vi "D-O Module (Main) Try Again.vi"(7 "Name of Parent Panel":string="Main.vi", 9 "New Center Coords":T1={"Horizontal"=470, "Vertical"=200}, 10 "Config":variant, 11 "Main UI Message Queue":refnum<queue>) -> ()   [LabVIEW 2018]
uses:
  support/Message Queue/Message Cluster.ctl
  <vilib>/Utility/miscctls.llb/LVPoint32TypeDef.ctl
  controls/UI State.ctl
  controls/UI Data.ctl
  D-O Module Config Cluster.ctl
  Valve Clusters.ctl
  D-O Module Settings Cluster.ctl
  D-O Device Settings Cluster.ctl
  VICI Electronic Actuator/VICI Electronic Actuator Settings.ctl
  D-O Module State Cluster.ctl
  Measure Instrument/State Enum.ctl
  D-O Module Display.ctl
  Sequencing/Squence Update Cluster.ctl
  support/Message Queue/Enqueue Message (Single).vi
  support/Message Queue/Message Queue.lvlib
  support/Support Library.lvlib
  support/Command Log VIs/Command Logging.lvlib
  D-O Module.lvlib
  Sequencing/Sequencing Library.lvlib
  Measure Instrument/Feed Module Engine.lvlib
  support/User Event - Stop/User Event - Stop.lvlib
  D-O Settings Dialog.vi
  Measure Instrument/D-O Module Engine.lvlib
  DIO Valve/VICI Electronic Actuator.lvlib
panel:
  out "Sequence Started":bool
  out "ScanCode":i16
  in  "Settings Button":bool
  in  "Exit":bool
  out "Ring":u16(ring)=2
  out "Status":string
  out "Log File path":path
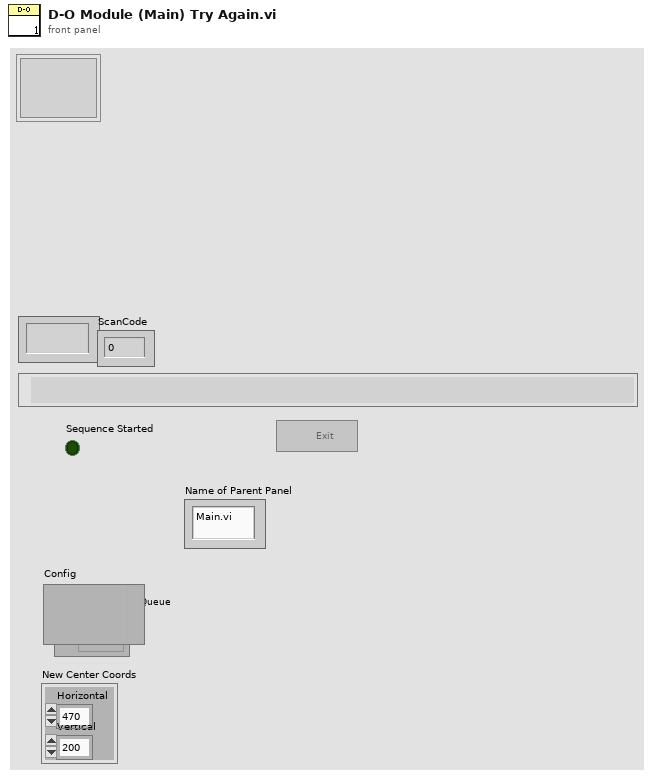
[diagram p1: front panel]
types:
  T1 = typedef "LVPoint32TypeDef.ctl" = cluster{"Horizontal":i32, "Vertical":i32}
  T2 = typedef "D-O Module.lvlib/D-O Module State Cluster.ctl" = cluster{"D-O Module Config":T3, "State":T8, "Start Time":timestamp, "Current Time":timestamp, "First Iteration":bool, "Data":cluster{"Valve State":T5}, "Process Name":string, "Queue Name":string, "Program On?":bool}
  T3 = typedef "D-O Module.lvlib/D-O Module Config Cluster.ctl" = cluster{"GUID":string, "Drop Coords":T1, "Process Name":string, "User name":string, "Queue Name":string, "Settings":T4, "Load Count":i32}
  T4 = typedef "D-O Module.lvlib/Valve Clusters.ctl" = cluster{"Valve Settings":T5, "Valve Type":enum16{"Default", "Digital Output Valve", "VICI Electronic Actuator"}, "Time On (Sec)":dbl, "Time Off (Sec)":dbl, "Run?":bool}
  T5 = typedef "D-O Module.lvlib/D-O Module Settings Cluster.ctl" = cluster{"D-O Settings":T6, "VICI Electronic Actuator":T7}
  T6 = typedef "D-O Module.lvlib/D-O Device Settings Cluster.ctl" = cluster{"DAQmx Task Name":refnum<k21>, "Output Channel":u16, "Output Channel Names":string[]}
  T7 = typedef "VICI Electronic Actuator.lvlib/VICI Electronic Actuator Settings.ctl" = cluster{"VISA resource name":refnum<visa-resource-name>, "Mode":enum16{"Two Positions With Stops", "Two Positions Without Stops", "Mutiposition"}, "Simulated":bool}
  T8 = typedef "Feed Module.lvlib/Feed Module Engine.lvlib/State Enum.ctl" = enum16{"Measuring", "Idle", "Paused"}
  T9 = typedef "UI Data.ctl" = cluster{"Start Ref":refnum<vi>, "Trigger Ref":refnum<vi>, "Stop Ref":refnum<vi>, "Settings Ref":refnum<vi>, "Status Ref":refnum<vi>, "Exit Ref":refnum<vi>, "Data Ref":refnum<vi>}
  T10 = typedef "UI State.ctl" = enum16{"Idle", "Acquiring and Logging", "Waiting for Exit", "Waiting for Exit (Acq Stopped)", "Waiting for Exit (Log Stopped)", "Waiting for Stop", "Waiting for Stop (Acq Stopped)", "Waiting for Stop (Log Stopped)"}
  T11 = typedef "D-O Module.lvlib/All Message Queues.ctl" = cluster{"Engine":refnum<queue>, "D-O UI":refnum<queue>, "D-O Engine":refnum<queue>, "D-O Display":refnum<queue>}
  T12 = typedef "Sequencing Library.lvlib/Squence Update Cluster.ctl" = cluster{"Auto?":bool, "Manual Entry":dbl, "Setpoint":dbl}
  T13 = enum8{"Enabled", "Disabled", "Disabled and Grayed Out"}
  T14 = typedef "D-O Module.lvlib/D-O Module Display.ctl" = cluster{"D-O State ":u16, "Cycle Period":dbl}
  T15 = cluster{"Shift":bool, "Ctrl":bool, "Alt":bool, "Cmd":bool, "Opt":bool}
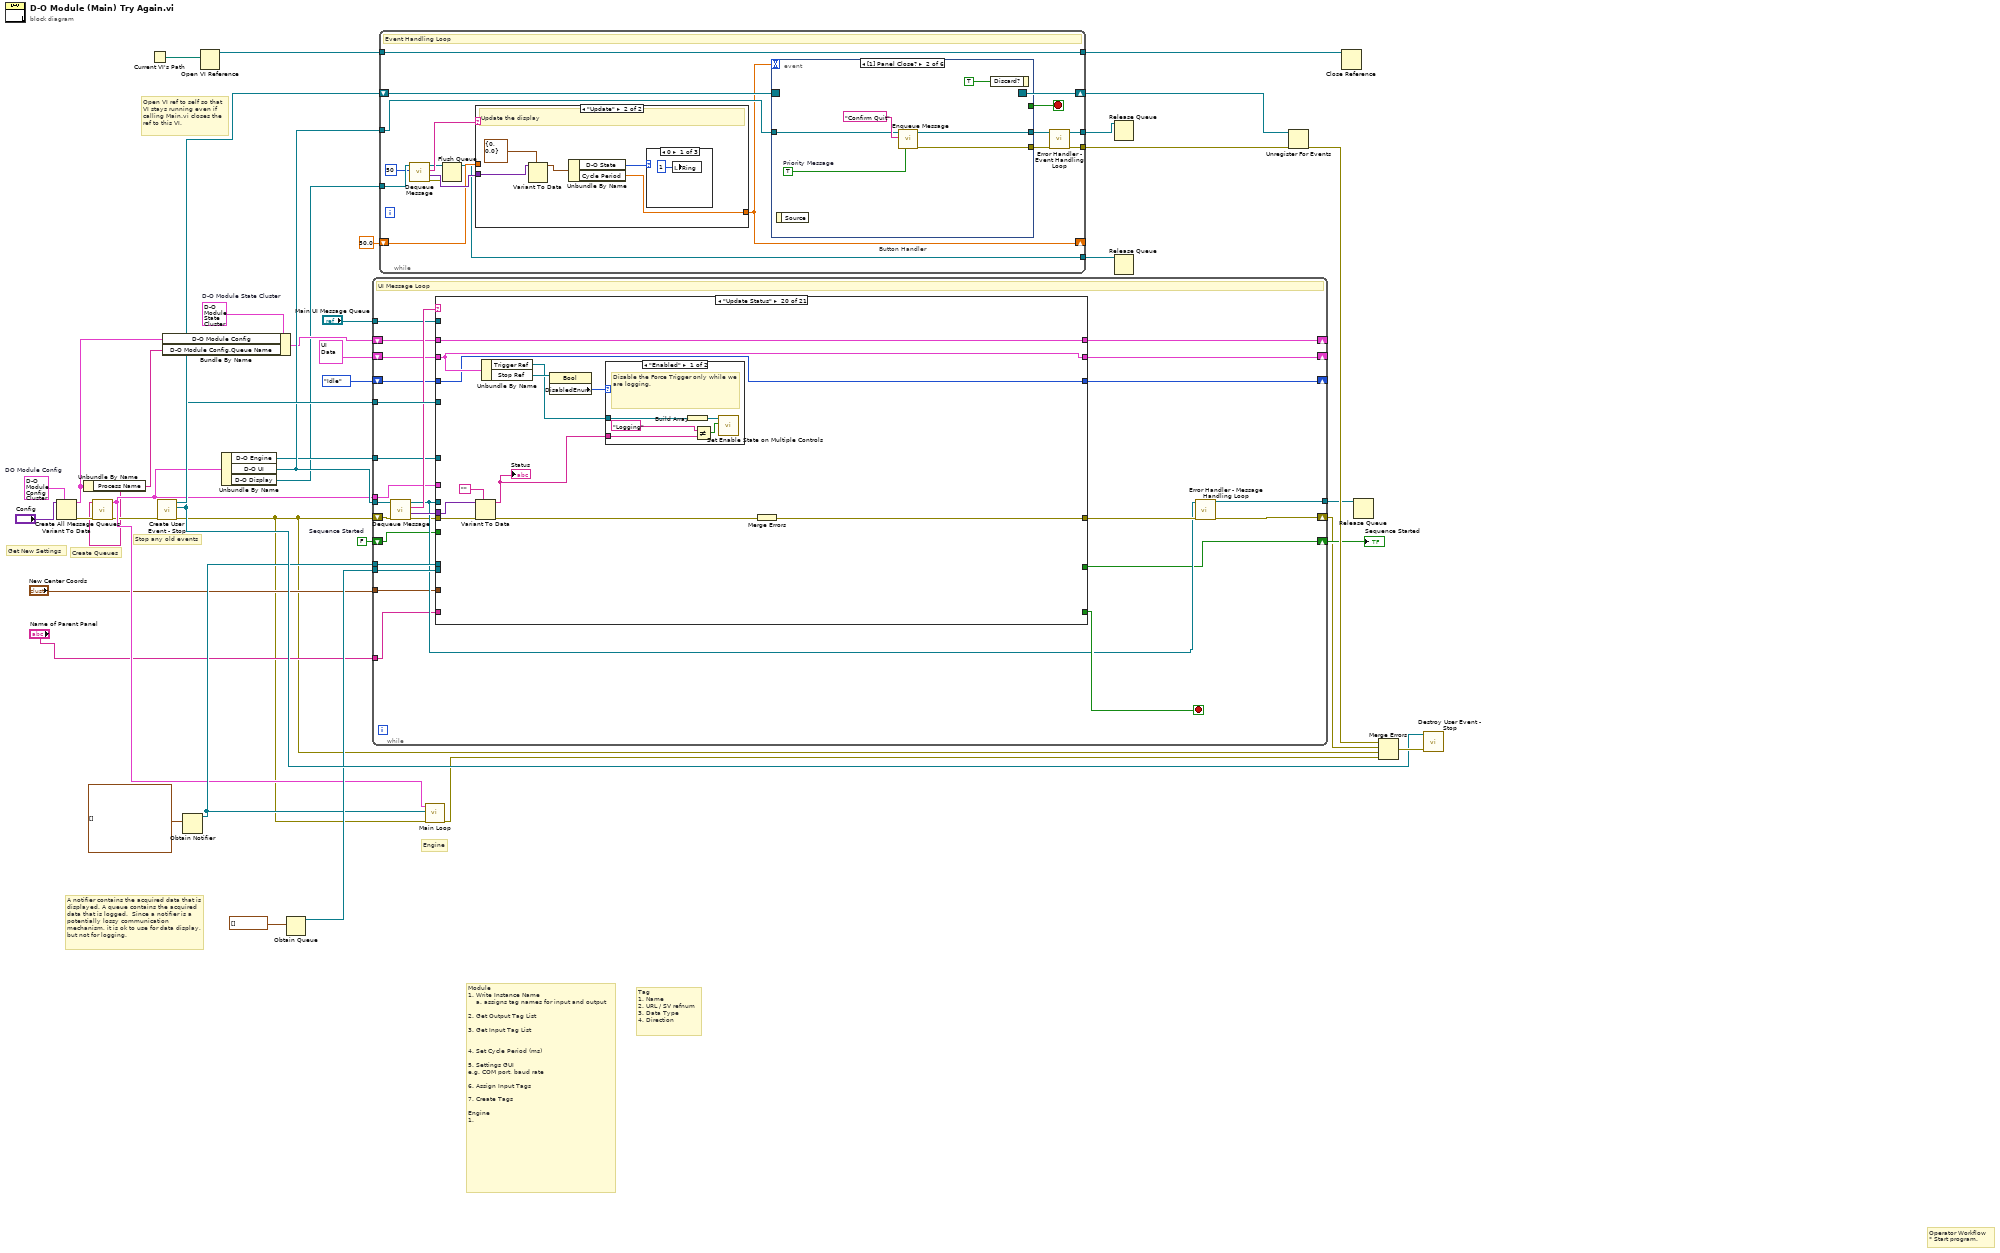
[diagram p0: block diagram]
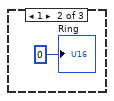
[diagram p3: hidden frame]
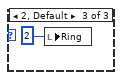
[diagram p4: hidden frame]
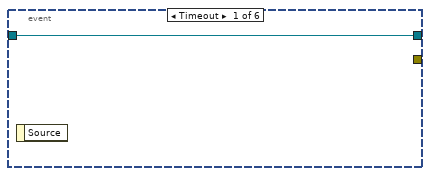
[diagram p5: hidden frame]
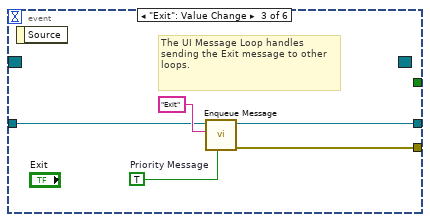
[diagram p6: hidden frame]
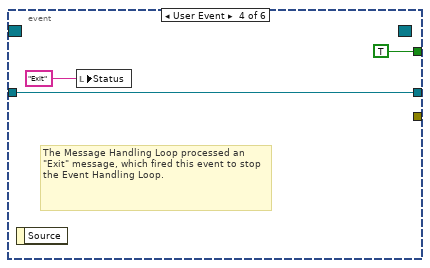
[diagram p7: hidden frame]
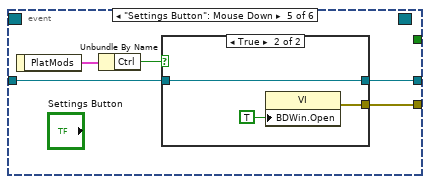
[diagram p8: hidden frame]
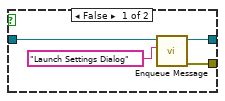
[diagram p9: hidden frame]
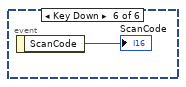
[diagram p10: hidden frame]
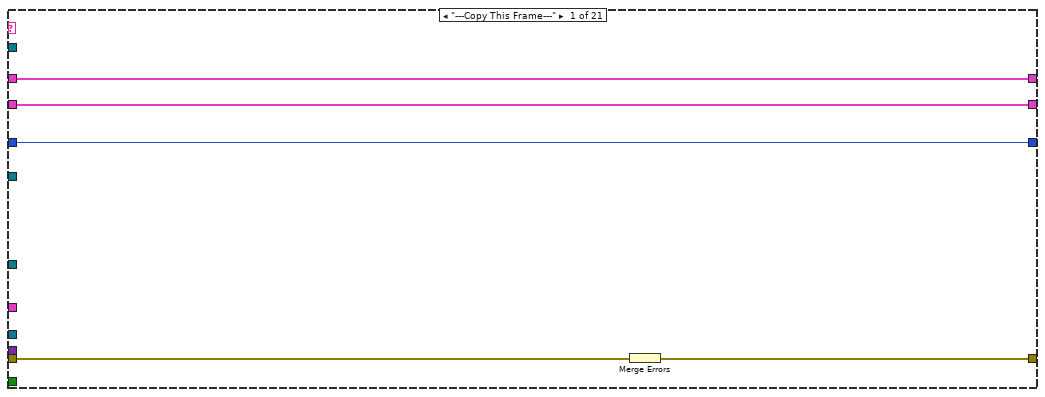
[diagram p11: hidden frame]
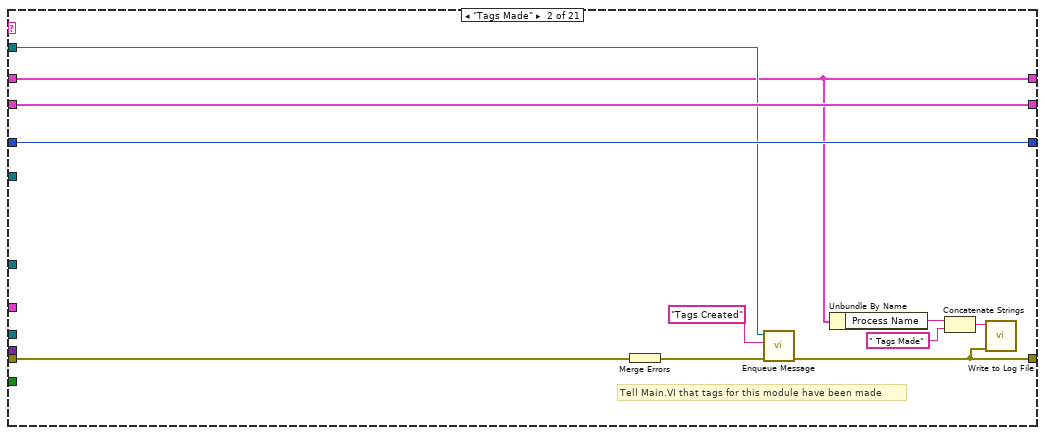
[diagram p12: hidden frame]
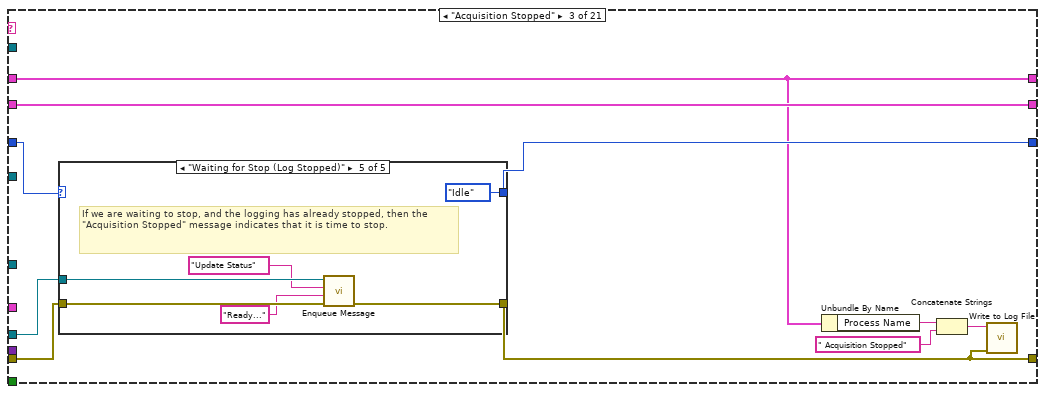
[diagram p13: hidden frame]
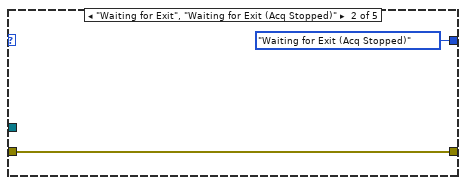
[diagram p15: hidden frame]
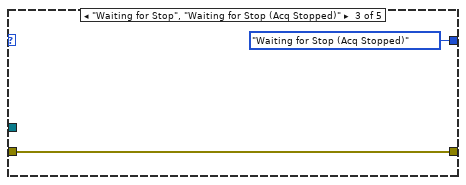
[diagram p16: hidden frame]
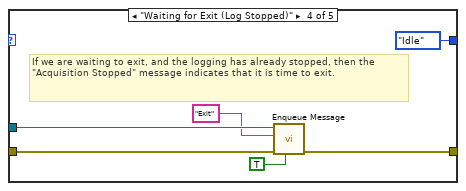
[diagram p17: hidden frame]
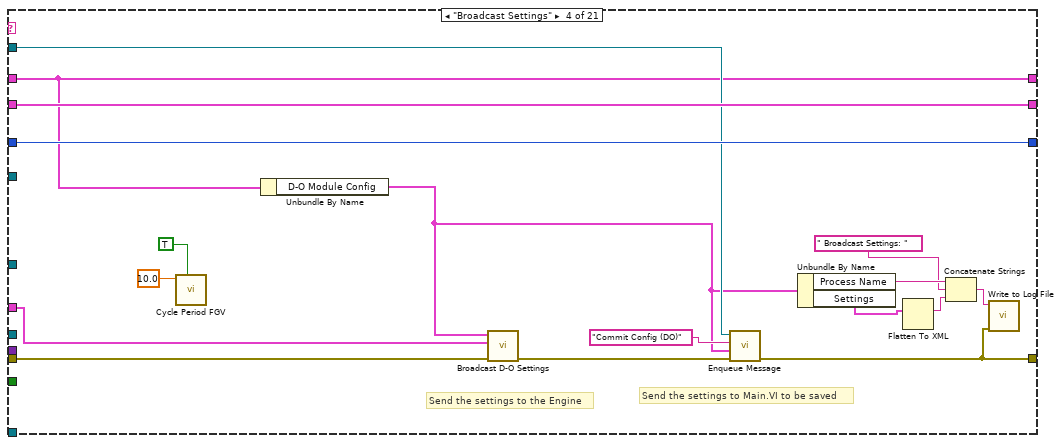
[diagram p18: hidden frame]
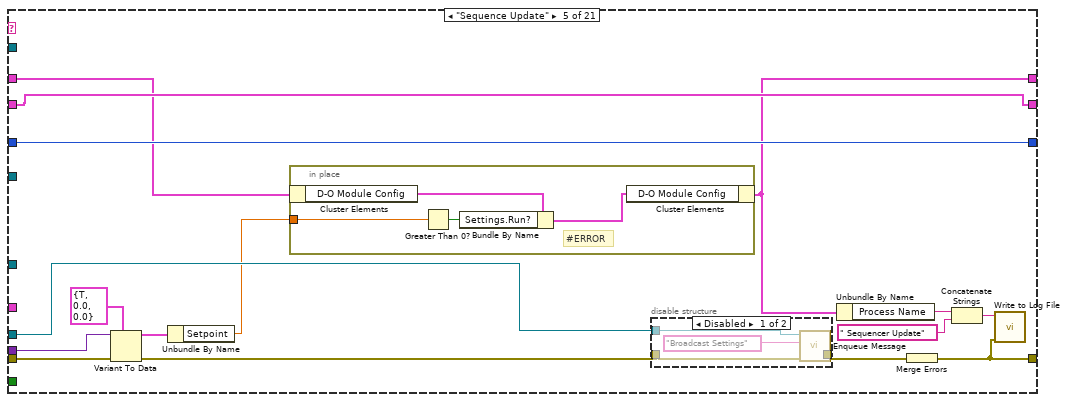
[diagram p19: hidden frame]
diagram:
  w19 = T2 {"D-O Module Config"={"GUID"="", "Drop Coords"={"Horizontal"=0, "Vertical"=0}, "Process Name"="", "User name"="", "Queue Name"="", "Settings"={"Valve Settings"={"D-O Settings"={"DAQmx Task Name"="", "Output Channel"=0, "Output Channel Names"=[]}, "VICI Electronic Actuator"={"VISA resource name"="", "Mode"=enum."Two Positions With Stops", "Simulated"=FALSE}}, "Valve Type"=enum."Digital Output Valve", "Time On (Sec)"=0.0, "Time Off (Sec)"=0.0, "Run?"=FALSE}, "Load Count"=0}, "State"=enum."Idle", "Start Time"=timestamp(0 s since 1904-01-01), "Current Time"=timestamp(0 s since 1904-01-01), "First Iteration"=FALSE, "Data"={"Valve State"={"D-O Settings"={"DAQmx Task Name"="", "Output Channel"=0, "Output Channel Names"=[]}, "VICI Electronic Actuator"={"VISA resource name"="", "Mode"=enum."Two Positions With Stops", "Simulated"=FALSE}}}, "Process Name"="", "Queue Name"="", "Program On?"=FALSE}  # D-O Module State Cluster
  w11 = T3 {"GUID"="", "Drop Coords"={"Horizontal"=0, "Vertical"=0}, "Process Name"="", "User name"="", "Queue Name"="", "Settings"={"Valve Settings"={"D-O Settings"={"DAQmx Task Name"="", "Output Channel"=0, "Output Channel Names"=[]}, "VICI Electronic Actuator"={"VISA resource name"="", "Mode"=enum."Two Positions With Stops", "Simulated"=FALSE}}, "Valve Type"=enum."Default", "Time On (Sec)"=0.0, "Time Off (Sec)"=0.0, "Run?"=FALSE}, "Load Count"=0}  # DO Module Config
  w12 = FALSE  # Sequence Started
  # "Stop any old events"
  # "Create Queues"
  # "Get New Settings"
  # "Open VI ref to self so that\nVI stays running even if\ncalling Main.vi closes the\nref to this VI."
  # "Engine"
  # "Operator Workflow\n* Start program."
  # "Module \n1. Write Instance Name\n    a. assigns tag names for input and output\n\n2. Get Output Tag List\n\n3. Get Input Tag List\n\n\n4. Set Cycle Period (ms)\n\n5. Settings GUI\ne.g. COM port, baud rate\n\n6. Assign Input Tags\n\n7. Create Tags\n\nEngine\n1."
  # "Tag\n1. Name\n2. URL / SV refnum\n3. Data Type\n4. Direction"
  # "A notifier contains the acquired data that is displayed. A queue contains the acquired data that is logged.  Since a notifier is a potentially lossy communication mechanism, it is ok to use for data display, but not for logging."
  n1 = Variant To Data(type=w11, Variant="Config") -> (data=w10:T3, error out=w9:errorcluster)  [unwired: 1 in]
  n2 = Unbundle By Name(w10) -> ("Process Name"=w6:string)
  n3 = call "Create All Message Queues.vi"("error in (no error)"=w9, "Process Name"=w6) -> ("error out"=w8:errorcluster, "Message Queues"=w16:T11)  [unwired: 8 in]
  n4 = Current VI's Path() -> (path=w22:path)
  n5 = call "Create User Event - Stop.vi"("error in (no error)"=w8) -> ("error out"=w7:errorcluster, "User Event - Stop"=w36:refnum<user-event>, "Stop Event Registration Refnum"=w37:refnum<event-registration>)  [unwired: 8 in]
  n6 = Bundle By Name(cluster=w19, "D-O Module Config"=w10, "D-O Module Config.Queue Name"=w6) -> (w21:T2)
  n7 = Obtain Notifier(notification data type=waveform(dbl)[] []) -> (notifier out=w25:refnum<notifier>)  [unwired: 3 in, 2 out]
  n8 = Open VI Reference(vi path=w22) -> (vi reference=w23:refnum<vi>)  [unwired: 5 in, 1 out]
  n9 = Unbundle By Name(w16) -> ("D-O Engine"=w28:refnum<queue>, "D-O UI"=w32:refnum<queue>, "D-O Display"=w18:refnum<queue>)
  n10 = Obtain Queue(element data type=waveform(dbl)[] []) -> (queue out=w27:refnum<queue>)  [unwired: 4 in, 2 out]
  n11 = while {
    tunnel: w32 -> [w60]
    tunnel: w36 -> [w64]
    shift-right: [w54] -> w2
    shift-left: w7 -> [w63]
    shift-right: [w41] -> _
    shift-left: w21 -> [w48]
    shift-right: [w58] -> _
    shift-left: T9 {"Start Ref"=refnum, "Trigger Ref"=refnum, "Stop Ref"=refnum, "Settings Ref"=refnum, "Status Ref"=refnum, "Exit Ref"=refnum, "Data Ref"=refnum} ("Measurement UI Controls") -> [w59]
    tunnel: w25 -> [w57]
    tunnel: w27 -> [w56]
    shift-right: [w51] -> _
    shift-left: UI_State."Idle" ("UI State") -> [w52]
    tunnel: w28 -> [w50]
    tunnel: "Main UI Message Queue" -> [w47]
    tunnel: w16 -> [w46]
    tunnel: "New Center Coords" -> [w45]
    tunnel: "Name of Parent Panel" -> [w44]
    shift-right: [w43] -> w13
    shift-left: w12 -> [w42]
    tunnel: [w40] -> w1
    stop <- w65 stop-if-true
    # "UI Message Loop"
    n12 = call "Dequeue Message.vi"("error in (no error)"=w63, "Message Queue"=w60) -> ("error out"=w49:errorcluster, "Message Data"=w61:variant, "Message"=w62:string, "dup Message Queue"=w53:refnum<queue>)  [unwired: 6 in]
    n13 = case "Message Cases" shown="\"Update Status\"" w62 {
      selector: w62 -> [_ _ _ _ _ _ _ _ _ _ _ _ _ _ _ _ _ _ _ _ w487]
      tunnel: w53 -> [_ _ w87 _ w139 w158 _ w216 w231 w258 _ w292 w311 w317 w353 w384 _ _ w444 _ _]
      tunnel: w49 -> [w70 w81 w88 w123 w138 w157 w184 w197 w235 w262 w277 w287 w309 w319 w351 w383 w410 w421 w446 w479 _]
      tunnel: [w69 w75 w86 w116 w129 w152 w185 w191 w225 w237 w277 w282 w305 w318 w342 w372 w414 w426 w441 w480 w486] -> w55
      tunnel: [_ _ _ _ _ _ _ _ _ TRUE _ _ _ _ _ _ _ _ _ _ _] -> w65
      tunnel: w61 -> [_ _ _ _ w140 _ w187 _ w234 w246 _ _ _ _ _ _ _ _ _ w478 _]
      tunnel: w64 -> [_ _ _ _ _ _ _ _ _ w261 _ _ _ _ _ _ _ _ _ _ _]
      tunnel: w48 -> [w66 w71 w82 w120 w128 w151 w182 w195 w222 w238 w268 w278 w300 w316 w347 w379 w408 w422 w448 w469 w492]
      tunnel: w59 -> [w68 w80 w91 w126 w141 w160 w189 w213 w236 w259 w276 w288 w313 w322 w348 w380 w413 w431 w464 w475 w497]
      tunnel: [w68 w80 w91 w126 w141 w160 w189 w213 w236 w259 w275 w288 w313 w322 w348 w380 w413 w431 w464 w475 w497] -> w58
      tunnel: w57 -> [_ _ _ _ _ _ _ _ _ w257 _ _ _ _ _ _ _ _ _ _ _]
      tunnel: w56 -> [_ _ _ _ _ _ _ _ _ w253 _ _ _ _ _ _ _ _ _ _ _]
      tunnel: w52 -> [w67 w79 w90 w125 w142 w159 w183 w202 w226 _ _ _ w312 w321 _ _ _ _ w453 w470 w496]
      tunnel: [w67 w79 w89 w125 w142 w156 w183 w203 w226 UI_State."Idle" ("UI State") UI_State."Idle" ("UI State") UI_State."Idle" ("UI State") w312 w320 UI_State."Acquiring and Logging" ("UI State") UI_State."Acquiring and Logging" ("UI State") UI_State."Acquiring and Logging" ("UI State") UI_State."Acquiring and Logging" ("UI State") w454 w470 w496] -> w51
      tunnel: w50 -> [_ _ _ _ _ _ _ w201 _ w245 _ _ _ _ _ _ w411 w429 w452 _ _]
      tunnel: w47 -> [_ w76 _ w122 _ _ _ _ _ w247 _ _ _ _ _ _ _ _ _ _ _]
      tunnel: [w66 w71 w82 w120 w127 w151 w182 w190 w222 w238 w268 w278 w301 w316 w341 w369 w408 w422 w437 w469 w492] -> w41
      tunnel: w46 -> [_ _ _ w118 _ _ _ _ _ _ _ _ w307 _ _ _ _ _ _ _ _]
      tunnel: w45 -> [_ _ _ _ _ _ _ _ _ _ _ w285 _ _ _ _ _ _ _ _ _]
      tunnel: w44 -> [_ _ _ _ _ _ _ _ _ _ _ w284 _ _ _ _ _ _ _ _ _]
      tunnel: [_ _ _ _ _ _ _ _ _ _ _ _ _ _ _ w377 _ _ _ _ _] -> w43
      tunnel: w42 -> [_ _ _ _ _ _ _ _ _ _ _ _ _ _ _ w373 _ _ _ _ _]
      frame "---Copy This Frame---" {
        # "Duplicate this frame when creating new messages.  Change this comment in the duplicated frame to describe this message."
        n14 = Merge Errors(w70) -> (w69:errorcluster)
      }
      frame "Tags Made" {
        # "Tell Main.VI that tags for this module have been made"
        # "Duplicate this frame when creating new messages.  Change this comment in the duplicated frame to describe this message."
        n15 = Merge Errors(w81) -> (w77:errorcluster)
        n16 = call-poly "Enqueue Message.vi"("error in (no error)"=w77, "Message"="Tags Created", "Message Queue"=w76) -> ("error out"=w75:errorcluster)  [unwired: 7 in, 1 out]
        n17 = Unbundle By Name(w71) -> ("Process Name"=w74:string)
        n18 = Concatenate Strings(w74, " Tags Made" ("text")) -> (w72:string)
        n19 = call "Write to Log File.vi"("error in"=w75, "text"=w72) -> ()  [unwired: 9 in, 1 out]
      }
      frame "Acquisition Stopped" {
        # "Logic for determining what action to take when the acquisition has stopped."
        n20 = case shown="\"Waiting for Stop (Log Stopped)\"" w90 {
          selector: w90 -> [w93 _ _ _ _]
          tunnel: [w93 UI_State."Waiting for Exit (Acq Stopped)" ("UI State") UI_State."Waiting for Stop (Acq Stopped)" ("UI State") UI_State."Idle" ("UI State") UI_State."Idle" ("UI State")] -> w89
          tunnel: w88 -> [w92 w94 w96 w102 w108]
          tunnel: [w92 w94 w96 w101 w107] -> w86
          tunnel: w87 -> [_ _ _ w100 w106]
          frame Default {
          }
          frame "Waiting for Exit", "Waiting for Exit (Acq Stopped)" {
          }
          frame "Waiting for Stop", "Waiting for Stop (Acq Stopped)" {
          }
          frame "Waiting for Exit (Log Stopped)" {
            # "If we are waiting to exit, and the logging has already stopped, then the \"Acquisition Stopped\" message indicates that it is time to exit."
            n21 = call-poly "Enqueue Message.vi"("Priority Message? (F)"=TRUE, "error in (no error)"=w102, "Message"="Exit", "Message Queue"=w100) -> ("error out"=w101:errorcluster)  [unwired: 6 in, 1 out]
          }
          frame "Waiting for Stop (Log Stopped)" {
            # "If we are waiting to stop, and the logging has already stopped, then the \"Acquisition Stopped\" message indicates that it is time to stop."
            n22 = call-poly "Enqueue Message.vi"("error in (no error)"=w108, "Message Data"="Ready..." ("Message"), "Message"="Update Status", "Message Queue"=w106) -> ("error out"=w107:errorcluster)  [unwired: 6 in, 1 out]
          }
        }
        n23 = Unbundle By Name(w82) -> ("Process Name"=w85:string)
        n24 = Concatenate Strings(w85, " Acquisition Stopped" ("text")) -> (w83:string)
        n25 = call "Write to Log File.vi"("error in"=w86, "text"=w83) -> ()  [unwired: 9 in, 1 out]
      }
      frame "Broadcast Settings" {
        # "Send the settings to Main.VI to be saved"
        # "Send the settings to the Engine"
        # "Send the 'Update Settings' message to the Logging and Acquisition message loops."
        n26 = call "Cycle Period FGV.vi"("Write"=TRUE, "Cycle Period In (ms)"=10.0) -> ()  [unwired: 8 in, 2 out]
        n27 = Unbundle By Name(w120) -> ("D-O Module Config"=w112:T3)
        n28 = call "Broadcast D-O Settings.vi"("error in (no error)"=w123, "Message Queues"=w118, "D-O Module Config"=w112) -> ("error out"=w121:errorcluster)  [unwired: 8 in]
        n29 = call-poly "Enqueue Message.vi"("error in (no error)"=w121, "Message Data"=w112, "Message"="Commit Config (DO)", "Message Queue"=w122) -> ("error out"=w116:errorcluster)  [unwired: 6 in, 1 out]
        n30 = Unbundle By Name(w112) -> ("Process Name"=w115:string, "Settings"=w110:T4)
        n31 = Flatten To XML(anything=w110) -> (xml string=w111:string)
        n32 = Concatenate Strings(w115, " Broadcast Settings: " ("text"), w111) -> (w113:string)
        n33 = call "Write to Log File.vi"("error in"=w116, "text"=w113) -> ()  [unwired: 9 in, 1 out]
      }
      frame "Sequence Update" {
        n34 = Variant To Data(error in=w138, type=T12 {"Auto?"=TRUE, "Manual Entry"=0.0, "Setpoint"=0.0} ("Cluster"), Variant=w140) -> (data=w136:T12, error out=w134:errorcluster)
        n35 = Unbundle By Name(w136) -> ("Setpoint"=w133:dbl)
        n36 = in-place {
          in-place-border: w133 -> [w149]
          # "#ERROR"
          n37 = in-place-cluster #1(w128) -> ("D-O Module Config"=w148:T3)
          n38 = Greater Than 0?(x=w149) -> (x > 0?=w150:bool)
          n39 = Bundle By Name(cluster=w148, "Settings.Run?"=w150) -> (w147:T3)
          n40 = in-place-cluster #1("D-O Module Config"=w147) -> (w127:T2)
        }
        n41 = disable-structure shown="Disabled" {
          disable-tunnel: w139 -> [w146 _]
          disable-tunnel: [w145 _] -> w135
          disable-tunnel: w134 -> [w143 _]
          frame Disabled {
            n42 = call-poly "Enqueue Message.vi"("error in (no error)"=w143, "Message"="Broadcast Settings", "Message Queue"=w146) -> ("error out"=w145:errorcluster)  [unwired: 7 in, 1 out]
          }
          frame Enabled {
          }
        }
        n43 = Unbundle By Name(w127) -> ("Process Name"=w132:string)
        n44 = Merge Errors(w135) -> (w129:errorcluster)
        n45 = Concatenate Strings(w132, " Sequencer Update" ("text")) -> (w130:string)
        n46 = call "Write to Log File.vi"("error in"=w129, "text"=w130) -> ()  [unwired: 9 in, 1 out]
      }
      frame "Confirm Quit" {
        # "Confirm Quit - Message that can confirm whether or not the user wants to exit the application."
        n47 = case shown="\"Acquiring and Logging\"" w159 {
          tunnel: w158 -> [w165 w171]
          tunnel: w157 -> [w164 w169]
          tunnel: [w161 w168] -> w152
          tunnel: [UI_State."Idle" ("UI State") w167] -> w156
          frame Default {
            # "If 'Confirm Quit' comes in while the system is idle, there is no need for a confirmation message."
            n48 = call-poly "Enqueue Message.vi"("Priority Message? (F)"=TRUE, "error in (no error)"=w164, "Message"="Exit", "Message Queue"=w165) -> ("error out"=w161:errorcluster)  [unwired: 6 in, 1 out]
          }
          frame "Acquiring and Logging" {
            n49 = Two Button Dialog(message="Are you sure you want to quit while the acquisition is running?" ("Confirm Quit Message"), 1:"No" ("No"), 2:"Yes" ("Yes")) -> (T button?=w170:bool)
            n50 = case shown="False" w170 {
              tunnel: w171 -> [_ w181]
              tunnel: w169 -> [w175 w180]
              tunnel: [w175 w179] -> w168
              tunnel: [UI_State."Acquiring and Logging" ("UI State") UI_State."Waiting for Exit" ("UI State")] -> w167
              frame False {
                # "User did not want to quit."
              }
              frame True {
                n51 = call-poly "Enqueue Message.vi"("error in (no error)"=w180, "Message"="Stop", "Message Queue"=w181) -> ("error out"=w179:errorcluster)  [unwired: 7 in, 1 out]
              }
            }
          }
        }
        n52 = Unbundle By Name(w151) -> ("Process Name"=w155:string)
        n53 = Concatenate Strings(w155, " Quit" ("text")) -> (w153:string)
        n54 = call "Write to Log File.vi"("error in"=w152, "text"=w153) -> ()  [unwired: 9 in, 1 out]
      }
      frame "Display Log File Path" {
        n55 = Variant To Data(error in=w184, type=path "", Variant=w187) -> (data=→"Log File path":path, error out=w185:errorcluster)
      }
      frame "E-Stop" {
        # "Pause the DO when E-Stop is sent"
        # "Message Acquisition and Logging loops to stop"
        # "Enable: Start, Exit, Settings\nDisable: Stop"
        # "Stop the pumps."
        n56 = Unbundle By Name(w213) -> ("Trigger Ref"=w204:refnum<vi>, "Stop Ref"=w205:refnum<vi>, "Start Ref"=w208:refnum<vi>, "Exit Ref"=w207:refnum<vi>, "Settings Ref"=w206:refnum<vi>)
        n57 = call-poly "Enqueue Message.vi"("error in (no error)"=w197, "Message Data"="Ready..." ("Ready..."), "Message"="Update Status", "Message Queue"=w216) -> ("error out"=w199:errorcluster)  [unwired: 6 in, 1 out]
        n58 = Build Array(w208, w207, w206) -> (w211:refnum<vi>[])
        n59 = Build Array(w204, w205) -> (w210:refnum<vi>[])
        n60 = call-poly "Enqueue Message.vi"("error in (no error)"=w199, "Message"="Pause", "Message Queue"=w201) -> ("error out"=w198:errorcluster)  [unwired: 7 in, 1 out]
        n61 = call "Set Enable State on Multiple Controls.vi"("Enable?"=FALSE, "Controls"=w210) -> ()  [unwired: 10 in]
        n62 = call "Set Enable State on Multiple Controls.vi"("Enable?"=TRUE, "Controls"=w211) -> ()  [unwired: 10 in]
        n63 = case shown="Default" w202 {
          selector: w202 -> [_ w218]
          tunnel: [UI_State."Waiting for Stop" ("UI State") w218] -> w203
          frame Default {
          }
          frame "Waiting for Exit" {
          }
        }
        n64 = Merge Errors(w198) -> (w191:errorcluster)
        n65 = Bundle By Name(cluster=w195, "State"=State_Enum."Idle") -> (w190:T2)
        n66 = Unbundle By Name(w190) -> ("Process Name"=w194:string)
        n67 = Concatenate Strings(w194, " E-STOP" ("text")) -> (w192:string)
        n68 = call "Write to Log File.vi"("error in"=w191, "text"=w192) -> ()  [unwired: 9 in, 1 out]
      }
      frame "Error" {
        # "Error - Check the error message data and respond accordingly. This message is sent by the \"Error Handler\" VIs at the end of each loop in this application."
        n69 = Variant To Data(error in=w235, type=errorcluster {"status"=FALSE, "code"=0, "source"=""} ("error out"), Variant=w234) -> (data=w232:errorcluster, error out=w228:errorcluster)
        n70 = call <vilib>:"Simple Error Handler.vi"("error in (no error)"=w232) -> ()  [unwired: 4 in, 5 out]
        n71 = call-poly "Enqueue Message.vi"("Priority Message? (F)"=TRUE, "Message"="Exit", "Message Queue"=w231) -> ("error out"=w227:errorcluster)  [unwired: 7 in, 1 out]
        n72 = Merge Errors(w227, w228) -> (w225:errorcluster)
        n73 = Unbundle By Name(w222) -> ("Process Name"=w224:string)
        n74 = call <vilib>:"General Error Handler.vi"("error in (no error)"=w225) -> ("message"=w220:string, "error out"=w219:errorcluster)  [unwired: 10 in, 3 out]
        n75 = Concatenate Strings(w224, " Error: " ("text"), w220) -> (w223:string)
        n76 = call "Write to Log File.vi"("error in"=w219, "text"=w223) -> ()  [unwired: 9 in, 1 out]
      }
      frame "Exit" {
        w250 = TRUE  # Delete Module?
        # "Stop DO Engine then Close it"
        # "Don't check the error outs. The acquisition and logging queues may have already been released."
        # "Close references owned by the Main VI."
        # "Stop the VI"
        # "Exit - Fire the User Event to stop the Event Handling Loop.  Also send Exit messages to the Acquisition and Logging loops."
        n77 = Release Queue(queue=w258, error in (no error)=w262) -> (error out=w256:errorcluster)  [unwired: 1 in, 2 out]
        n78 = call "Fire User Event - Stop.vi"("User Event - Stop"=w261) -> ("error out"=w260:errorcluster)  [unwired: 10 in]
        n79 = Release Notifier(notifier=w257, error in (no error)=w256) -> (error out=w255:errorcluster)  [unwired: 1 in, 2 out]
        n80 = Release Queue(queue=w253, error in (no error)=w255) -> (error out=w254:errorcluster)  [unwired: 1 in, 2 out]
        n81 = call-poly "Enqueue Message.vi"("Message"="Stop", "Message Queue"=w245) -> ("dup Message Queue"=w243:refnum<queue>)  [unwired: 8 in, 1 out]
        n82 = Variant To Data(type=w250, Variant=w246) -> (data=w249:bool, error out=w251:errorcluster)  [unwired: 1 in]
        n83 = Select(t=w250, s=w251, f=w249) -> (s? t:f=w248:bool)
        n84 = call-poly "Enqueue Message.vi"("Message"="Exit", "Message Queue"=w243) -> ()  [unwired: 8 in, 2 out]
        n85 = case "Don't enqueue Delete Module if opening campaign because it\nwill already have been deleted and new config loaded and we create\na race condition." shown="True" w248 {
          tunnel: w247 -> [_ w266]
          tunnel: w238 -> [_ w265]
          frame False {
          }
          frame True {
            n86 = Unbundle By Name(w265) -> ("D-O Module Config.GUID"=w264:string)
            n87 = call-poly "Enqueue Message.vi"("Message Data"=w264, "Message"="Delete Module", "Message Queue"=w266) -> ()  [unwired: 7 in, 2 out]
          }
        }
        n88 = Merge Errors(w260, w254) -> (w237:errorcluster)
        n89 = Unbundle By Name(w238) -> ("Process Name"=w241:string)
        n90 = Concatenate Strings(w241, " Exit" ("text")) -> (w239:string)
        n91 = call "Write to Log File.vi"("error in"=w237, "text"=w239) -> ()  [unwired: 9 in, 1 out]
      }
      frame "Init UI Refs" {
        # "Enable: Start, Exit, Settings\nDisable: Stop"
        # "Init UI Refs - Store control references for UI controls.  Also enable/disable controls appropriately."
        n92 = property class="VI"("Front Panel.Closeable"=TRUE ("Front Panel Window:Closeable")) -> ()  [unwired: 2 in, 2 out]
        n93 = control-ref of="Status"() -> (w273:refnum<vi>)
        n94 = control-ref of="Exit"() -> (w270:refnum<vi>)
        n95 = Bundle By Name(cluster=w276, "Status Ref"=w273, "Exit Ref"=w270) -> (w275:T9)
        n96 = Build Array(w270) -> (w272:refnum<vi>[])
        n97 = call "Set Enable State on Multiple Controls.vi"("Enable?"=TRUE, "Controls"=w272) -> ()  [unwired: 10 in]
      }
      frame "Initialize" {
        # "Initialize - Get configuration settings, then message the UI to initialize, and broadcast the settings to the other message loops."
        n98 = Unbundle By Name(w278) -> ("Process Name"=w283:string)
        n99 = property class="VI" props=["FP.State"]() -> (reference out=w286:refnum<vi>)  [unwired: 2 in, 2 out]
        n100 = call-poly "Enqueue Message.vi"("error in (no error)"=w287, "Message"="Init UI Refs", "Message Queue"=w292) -> ("error out"=w290:errorcluster, "dup Message Queue"=w291:refnum<queue>)  [unwired: 7 in]
        n101 = call "Make Child and Move.vi"("Process Name"=w283, "Name of Parent Panel"=w284, "New Center Coords"=w285, "VI in"=w286) -> ()  [unwired: 8 in]
        n102 = call-poly "Enqueue Message.vi"("error in (no error)"=w290, "Message"="Broadcast Settings", "Message Queue"=w291) -> ("error out"=w298:errorcluster, "dup Message Queue"=w297:refnum<queue>)  [unwired: 7 in]
        n103 = call-poly "Enqueue Message.vi"("error in (no error)"=w298, "Message Data"="Ready..." ("Ready..."), "Message"="Update Status", "Message Queue"=w297) -> ("error out"=w282:errorcluster)  [unwired: 6 in, 1 out]
        n104 = Unbundle By Name(w278) -> ("Process Name"=w281:string)
        n105 = Concatenate Strings(w281, " Initialize" ("text")) -> (w279:string)
        n106 = call "Write to Log File.vi"("error in"=w282, "text"=w279) -> ()  [unwired: 9 in, 1 out]
      }
      frame "Launch Settings Dialog" {
        # "Keep track of whether the Dialog has been opened."
        # "Launch the Settings Dialog when the user clicks the 'Settings' button."
        n107 = in-place {
          n108 = in-place-cluster #2(w300) -> ("D-O Module Config.Load Count"=w315:i32)
          n109 = Increment(x=w315) -> (x+1=w314:i32)
          n110 = in-place-cluster #2("D-O Module Config.Load Count"=w314) -> (w299:T2)
        }
        n111 = call-by-ref "?"("error in (no error)"=w309, "Message Queues"=w307, "D-O Module State Cluster In"=w299) -> ("error out"=w306:errorcluster, "D-O Module Config Out"=w308:T3)  [unwired: 7 in, 4 out]
        n112 = Bundle By Name(cluster=w300, "D-O Module Config"=w308) -> (w301:T2)
        n113 = call-poly "Enqueue Message.vi"("error in (no error)"=w306, "Message"="Broadcast Settings", "Message Queue"=w311) -> ("error out"=w305:errorcluster)  [unwired: 7 in, 1 out]
        n114 = Unbundle By Name(w301) -> ("Process Name"=w304:string)
        n115 = Concatenate Strings(w304, "Launch Settings Dialog" ("text")) -> (w302:string)
        n116 = call "Write to Log File.vi"("error in"=w305, "text"=w302) -> ()  [unwired: 9 in, 1 out]
      }
      frame "Logging Stopped" {
        # "Logic for determining what action to take when the logging has stopped."
        n117 = case shown="\"Waiting for Stop (Acq Stopped)\"" w321 {
          selector: w321 -> [w324 _ _ _ _]
          tunnel: [w324 UI_State."Waiting for Exit (Log Stopped)" ("UI State") UI_State."Waiting for Stop (Log Stopped)" ("UI State") UI_State."Idle" ("UI State") UI_State."Idle" ("UI State")] -> w320
          tunnel: w319 -> [w323 w325 w327 w333 w339]
          tunnel: [w323 w325 w327 w332 w338] -> w318
          tunnel: w317 -> [_ _ _ w331 w337]
          frame Default {
          }
          frame "Waiting for Exit", "Waiting for Exit (Log Stopped)" {
          }
          frame "Waiting for Stop", "Waiting for Stop (Log Stopped)" {
          }
          frame "Waiting for Exit (Acq Stopped)" {
            # "If we are waiting to exit, and the acquisition has already stopped, then the \"Logging Stopped\" message indicates that it is time to exit."
            n118 = call-poly "Enqueue Message.vi"("Priority Message? (F)"=TRUE, "error in (no error)"=w333, "Message"="Exit", "Message Queue"=w331) -> ("error out"=w332:errorcluster)  [unwired: 6 in, 1 out]
          }
          frame "Waiting for Stop (Acq Stopped)" {
            # "If we are waiting to stop, and the acquisition has already stopped, then the \"Logging Stopped\" message indicates that it is time to stop."
            n119 = call-poly "Enqueue Message.vi"("error in (no error)"=w339, "Message Data"="Ready..." ("Message"), "Message"="Update Status", "Message Queue"=w337) -> ("error out"=w338:errorcluster)  [unwired: 6 in, 1 out]
          }
        }
      }
      frame "Start" {
        # "Start the loops. In this case we could\n just do a straight start since there is \nonly one loop"
        # "Clear chart"
        # "Message Acquisition and Logging loops to start"
        # "Enable: Stop\nDisable: Start, Exit, Settings"
        # "Start - Enable/Disable buttons appropriately for an acquisition that has started, and update status display."
        n120 = Unbundle By Name(w348) -> ("Trigger Ref"=w359:refnum<vi>, "Stop Ref"=w360:refnum<vi>, "Start Ref"=w363:refnum<vi>, "Exit Ref"=w362:refnum<vi>, "Settings Ref"=w361:refnum<vi>, "Data Ref"=w350:refnum<vi>)
        n121 = property class="WFChart (strict)"(reference=w350, "History Data"=waveform(dbl)[][] []) -> ()  [unwired: 1 in, 2 out]
        n122 = Build Array(w363, w362, w361) -> (w366:refnum<vi>[])
        n123 = Build Array(w359, w360) -> (w365:refnum<vi>[])
        n124 = call-poly "Enqueue Message.vi"("error in (no error)"=w351, "Message"="Broadcast settings", "Message Queue"=w353) -> ("error out"=w354:errorcluster, "dup Message Queue"=w352:refnum<queue>)  [unwired: 7 in]
        n125 = call "Set Enable State on Multiple Controls.vi"("Enable?"=TRUE, "Controls"=w365) -> ()  [unwired: 10 in]
        n126 = call "Set Enable State on Multiple Controls.vi"("Enable?"=FALSE, "Controls"=w366) -> ()  [unwired: 10 in]
        n127 = call-poly "Enqueue Message.vi"("error in (no error)"=w354, "Message"="Start Loops", "Message Queue"=w352) -> ("error out"=w355:errorcluster)  [unwired: 7 in, 1 out]
        n128 = Merge Errors(w355) -> (w342:errorcluster)
        n129 = Bundle By Name(cluster=w347, "State"=State_Enum."Measuring") -> (w341:T2)
        n130 = Unbundle By Name(w341) -> ("Process Name"=w345:string)
        n131 = Concatenate Strings(w345, " Start" ("text")) -> (w343:string)
        n132 = call "Write to Log File.vi"("error in"=w342, "text"=w343) -> ()  [unwired: 9 in, 1 out]
      }
      frame "Sequence Start" {
        # "Clear chart"
        # "Message Acquisition and Logging loops to start"
        # "Enable: Stop\nDisable: Start, Exit, Settings"
        # "Start - Enable/Disable buttons appropriately for an acquisition that has started, and update status display."
        n133 = Unbundle By Name(w380) -> ("Trigger Ref"=w387:refnum<vi>, "Stop Ref"=w388:refnum<vi>, "Start Ref"=w391:refnum<vi>, "Exit Ref"=w390:refnum<vi>, "Settings Ref"=w389:refnum<vi>, "Data Ref"=w382:refnum<vi>)
        n134 = property class="WFChart (strict)"(reference=w382, "History Data"=waveform(dbl)[][] []) -> ()  [unwired: 1 in, 2 out]
        n135 = Build Array(w391, w390, w389) -> (w394:refnum<vi>[])
        n136 = Build Array(w387, w388) -> (w393:refnum<vi>[])
        n137 = call-poly "Enqueue Message.vi"("error in (no error)"=w383, "Message"="Broadcast settings", "Message Queue"=w384) -> ("error out"=w376:errorcluster, "dup Message Queue"=w375:refnum<queue>)  [unwired: 7 in]
        n138 = call "Set Enable State on Multiple Controls.vi"("Enable?"=TRUE, "Controls"=w393) -> ()  [unwired: 10 in]
        n139 = call "Set Enable State on Multiple Controls.vi"("Enable?"=FALSE, "Controls"=w394) -> ()  [unwired: 10 in]
        n140 = case shown="False" w373 {
          selector: w373 -> [_ w401]
          tunnel: [w400 w401] -> w377
          tunnel: w376 -> [w399 w402]
          tunnel: w375 -> [w397 _]
          tunnel: [w396 w402] -> w374
          frame False {
            w400 = TRUE  # Sequence Started
            # "Start the loops. In this case we could\n just do a straight start since there is \nonly one loop"
            # "Start the sequence loops"
            n141 = call-poly "Enqueue Message.vi"("error in (no error)"=w399, "Message"="Start Loops", "Message Queue"=w397) -> ("error out"=w396:errorcluster)  [unwired: 7 in, 1 out]
          }
          frame True {
            # "Sequence already started"
          }
        }
        n142 = Merge Errors(w374) -> (w372:errorcluster)
        n143 = Bundle By Name(cluster=w379, "State"=State_Enum."Measuring") -> (w369:T2)
        n144 = Unbundle By Name(w369) -> ("Process Name"=w371:string)
        n145 = Concatenate Strings(w371, " Sequence Start" ("text")) -> (w368:string)
        n146 = call "Write to Log File.vi"("error in"=w372, "text"=w368) -> ()  [unwired: 9 in, 1 out]
      }
      frame "Start Loops" {
        # "Start gets us going"
        # "Message Acquisition and Logging loops to start"
        # "Start - Enable/Disable buttons appropriately for an acquisition that has started, and update status display."
        n147 = Unbundle By Name(w408) -> ("D-O Module Config.Process Name"=w409:string, "D-O Module Config.Settings.Run?"=w403:bool)
        n148 = property class="VI"("Front Panel.Title"=w409) -> ()  [unwired: 2 in, 2 out]
        n149 = call-poly "Enqueue Message.vi"("error in (no error)"=w410, "Message Data"=w409, "Message"="Start", "Message Queue"=w411) -> ("error out"=w406:errorcluster, "dup Message Queue"=w404:refnum<queue>)  [unwired: 6 in]
        n150 = case shown="False" w403 {
          tunnel: w406 -> [w417 w419]
          tunnel: [w416 w419] -> w405
          tunnel: w404 -> [w415 _]
          frame False {
            # "If we are supposed to be paused we pause immediatly"
            n151 = call-poly "Enqueue Message.vi"("error in (no error)"=w417, "Message"="Pause", "Message Queue"=w415) -> ("error out"=w416:errorcluster)  [unwired: 7 in, 1 out]
          }
          frame True {
          }
        }
        n152 = Merge Errors(w405) -> (w414:errorcluster)
      }
      frame "Start Log" {
        # "Message Acquisition and Logging loops to start"
        # "Start - Enable/Disable buttons appropriately for an acquisition that has started, and update status display."
        n153 = Unbundle By Name(w422) -> ("D-O Module Config.Process Name"=w427:string)
        n154 = Build Array(w429) -> (w428:refnum<queue>[])
        n155 = for {
          tunnel: w421 -> [w435]
          tunnel: [w434] -> w420 mode=indexing
          tunnel: w428 -> [w433] mode=indexing
          tunnel: w427 -> [w432]
          n156 = call-poly "Enqueue Message.vi"("error in (no error)"=w435, "Message Data"=w432, "Message"="Start Log", "Message Queue"=w433) -> ("error out"=w434:errorcluster)  [unwired: 6 in, 1 out]
        }
        n157 = property class="VI"("Front Panel.Title"=w427) -> ()  [unwired: 2 in, 2 out]
        n158 = Merge Errors(w421, w420) -> (w426:errorcluster)
        n159 = Unbundle By Name(w422) -> ("Process Name"=w425:string)
        n160 = Concatenate Strings(w425, " Log Started" ("text")) -> (w423:string)
        n161 = call "Write to Log File.vi"("error in"=w426, "text"=w423) -> ()  [unwired: 9 in, 1 out]
      }
      frame "Stop" {
        # "Stop Pauses"
        # "Enable: Start, Exit, Settings\nDisable: Stop"
        # "Stop - Enable/Disable buttons appropriately for an acquisition that has stopped, and update status display."
        n162 = Unbundle By Name(w464) -> ("Trigger Ref"=w455:refnum<vi>, "Stop Ref"=w456:refnum<vi>, "Start Ref"=w459:refnum<vi>, "Exit Ref"=w458:refnum<vi>, "Settings Ref"=w457:refnum<vi>)
        n163 = call-poly "Enqueue Message.vi"("error in (no error)"=w446, "Message"="Broadcast settings", "Message Queue"=w444) -> ("error out"=w445:errorcluster, "dup Message Queue"=w443:refnum<queue>)  [unwired: 7 in]
        n164 = Build Array(w459, w458, w457) -> (w462:refnum<vi>[])
        n165 = Build Array(w455, w456) -> (w461:refnum<vi>[])
        n166 = call-poly "Enqueue Message.vi"("error in (no error)"=w445, "Message Data"="Ready..." ("Ready..."), "Message"="Update Status", "Message Queue"=w443) -> ("error out"=w451:errorcluster)  [unwired: 6 in, 1 out]
        n167 = call "Set Enable State on Multiple Controls.vi"("Enable?"=FALSE, "Controls"=w461) -> ()  [unwired: 10 in]
        n168 = call "Set Enable State on Multiple Controls.vi"("Enable?"=TRUE, "Controls"=w462) -> ()  [unwired: 10 in]
        n169 = call-poly "Enqueue Message.vi"("error in (no error)"=w451, "Message"="Pause", "Message Queue"=w452) -> ("error out"=w449:errorcluster)  [unwired: 7 in, 1 out]
        n170 = case shown="\"Waiting for Exit\"" w453 {
          selector: w453 -> [_ w468]
          tunnel: [UI_State."Waiting for Stop" ("UI State") w468] -> w454
          frame Default {
          }
          frame "Waiting for Exit" {
          }
        }
        n171 = Merge Errors(w449) -> (w441:errorcluster)
        n172 = Bundle By Name(cluster=w448, "State"=State_Enum."Paused") -> (w437:T2)
        n173 = Unbundle By Name(w437) -> ("Process Name"=w440:string)
        n174 = Concatenate Strings(w440, " Stopped" ("text")) -> (w438:string)
        n175 = call "Write to Log File.vi"("error in"=w441, "text"=w438) -> ()  [unwired: 9 in, 1 out]
      }
      frame "Update Status" {
        # "Update Display - Convert the message data to a string to display in the Status indicator."
        n176 = Variant To Data(error in=w479, type="", Variant=w478) -> (data=w472:string, error out=w476:errorcluster)
        "Status" <- w472
        n177 = Unbundle By Name(w475) -> ("Trigger Ref"=w471:refnum<vi>, "Stop Ref"=w474:refnum<vi>)
        n178 = property class="Bool"(reference=w474) -> ("DisabledEnum"=w473:T13)  [unwired: 1 in, 2 out]
        n179 = case shown="\"Enabled\"" w473 {
          tunnel: w472 -> [w483 _]
          tunnel: w471 -> [w484 _]
          frame "Enabled" {
            # "Disable the Force Trigger only while we are logging."
            n180 = Build Array(w484) -> (w485:refnum<vi>[])
            n181 = Not Equal?(x="Logging" ("Logging"), y=w483) -> (x != y?=w481:bool)
            n182 = call "Set Enable State on Multiple Controls.vi"("Enable?"=w481, "Controls"=w485) -> ()  [unwired: 10 in]
          }
          frame "Disabled", Default {
          }
        }
        n183 = Merge Errors(w476) -> (w480:errorcluster)
      }
      frame Default {
        # "'Default' case only runs if there is a message that isn't defined in any of the other cases.  Output a programming error."
        n184 = Concatenate Strings("The invalid message string " ("string"), w487, " was received in D-O Main." ("string")) -> (w488:string)
        n185 = Bundle By Name(cluster=errorcluster {"status"=TRUE, "code"=1, "source"=""} ("error constant"), "source"=w488) -> (w486:errorcluster)
        n186 = Unbundle By Name(w492) -> ("Process Name"=w495:string)
        n187 = Concatenate Strings(w495, " Invalid Message " ("text"), w487) -> (w493:string)
        n188 = call "Write to Log File.vi"("error in"=w486, "text"=w493) -> ()  [unwired: 9 in, 1 out]
      }
    }
    n189 = call "Error Handler - Message Handling Loop.vi"("error in (no error)"=w55, "Message Queue"=w53) -> ("dup error in"=w54:errorcluster, "dup Message Queue"=w40:refnum<queue>)  [unwired: 8 in]
  }
  "Sequence Started" <- w13
  n190 = while {
    tunnel: w32 -> [w509]
    tunnel: [w511] -> w39
    shift-right: [w510] -> w34
    shift-left: w37 -> [w515]
    tunnel: [w508] -> w24
    tunnel: w23 -> [w508]
    tunnel: w18 -> [w507]
    shift-right: [w504] -> _
    shift-left: 50.0 ("Cycle Period") -> [w503]
    tunnel: [w499] -> w4
    tunnel: [w498] -> w3
    stop <- w514 stop-if-true
    # "Event Handling Loop"
    n191 = call "Dequeue Message.vi"("timeout in ms (-1)"=50, "Message Queue"=w507) -> ("error out"=w500:errorcluster, "Message Data"=w505:variant, "Message"=w506:string, "dup Message Queue"=w501:refnum<queue>)  [unwired: 6 in]
    n192 = Flush Queue(queue=w501, error in (no error)=w500) -> (queue out=w498:refnum<queue>)  [unwired: 2 out]
    n193 = case shown="\"Update\"" w506 {
      tunnel: w505 -> [_ w521]
      tunnel: [w516 w517] -> w504
      tunnel: w503 -> [w516 _]
      frame "False", Default {
      }
      frame "Update" {
        # "Update the display"
        n194 = Variant To Data(type=T14 {"D-O State "=0, "Cycle Period"=0.0} ("FM Display"), Variant=w521) -> (data=w520:T14)  [unwired: 1 in, 1 out]
        n195 = Unbundle By Name(w520) -> ("D-O State"=w519:u16, "Cycle Period"=w517:dbl)
        n196 = case shown="0" w519 {
          frame 0 {
            n197 = local write "Ring"(u16 1 ("Ring")) -> ()
          }
          frame 1 {
            "Ring" <- u16 0 ("Ring")
          }
          frame 2, Default {
            n198 = local write "Ring"(u16 2 ("Ring")) -> ()
          }
        }
      }
    }
    n199 = event "Button Handler" shown="[1] Panel Close?" {
      selector: w515 -> [_ _ _ _ _ _]
      dyn-events: [_ _ _ _ _ _] -> w510
      timeout: w504 -> [_ _ _ _ _ _]
      tunnel: [_ _ _ TRUE ("Discard?") _ _] -> w514
      tunnel: w509 -> [w525 w528 w533 w537 w542 _]
      tunnel: [_ w526 w536 _ w544 _] -> w512
      tunnel: [w525 w527 w532 w537 w543 _] -> w513
      event Timeout {
        n200 = event-data() -> ()  [unwired: 1 in, 1 out]
      }
      event Panel Close? {
        w529 = TRUE  # Priority Message
        n201 = event-data() -> ()  [unwired: 1 in, 1 out]
        n202 = call-poly "Enqueue Message.vi"("Priority Message? (F)"=w529, "Message"="Confirm Quit", "Message Queue"=w528) -> ("error out"=w526:errorcluster, "dup Message Queue"=w527:refnum<queue>)  [unwired: 7 in]
        n203 = event-data("Discard?"=TRUE) -> ()  [unwired: 1 in, 1 out]
      }
      event "Exit": Value Change {
        w534 = TRUE  # Priority Message
        # "The UI Message Loop handles sending the Exit message to other loops."
        n204 = event-data() -> ()  [unwired: 1 in, 1 out]
        n205 = call-poly "Enqueue Message.vi"("Priority Message? (F)"=w534, "Message"="Exit", "Message Queue"=w533) -> ("error out"=w536:errorcluster, "dup Message Queue"=w532:refnum<queue>)  [unwired: 7 in]
      }
      event User Event {
        # "The Message Handling Loop processed an \"Exit\" message, which fired this event to stop the Event Handling Loop."
        n206 = event-data() -> ()  [unwired: 1 in, 1 out]
        n207 = local write "Status"("Exit" ("Exit String")) -> ()
      }
      event "Settings Button": Mouse Down {
        n208 = event-data() -> ("PlatMods"=w541:T15)  [unwired: 1 in]
        n209 = Unbundle By Name(w541) -> ("Ctrl"=w540:bool)
        n210 = case shown="True" w540 {
          tunnel: [w548 w549] -> w544
          tunnel: [w547 w550] -> w543
          tunnel: w542 -> [w546 w550]
          frame False {
            n211 = call-poly "Enqueue Message.vi"("Message"="Launch Settings Dialog", "Message Queue"=w546) -> ("error out"=w548:errorcluster, "dup Message Queue"=w547:refnum<queue>)  [unwired: 8 in]
          }
          frame True {
            n212 = property class="VI"("BDWin.Open"=TRUE ("Block Diagram Window:Open")) -> (error out=w549:errorcluster)  [unwired: 2 in, 1 out]
          }
        }
      }
      event Key Down {
        n213 = event-data() -> ("ScanCode"=→"ScanCode":i16)  [unwired: 1 in]
      }
    }
    n214 = call "Error Handler - Event Handling Loop.vi"("error in (no error)"=w512, "Message Queue"=w513) -> ("dup error in"=w511:errorcluster, "dup Message Queue"=w499:refnum<queue>)  [unwired: 8 in]
  }
  n215 = call "Main Loop.vi"("error in (no error)"=w7, "Chart Notifier"=w25, "Message Queues"=w16) -> ("error out"=w26:errorcluster)  [unwired: 8 in]
  n216 = Release Queue(queue=w4) -> ()  [unwired: 2 in, 3 out]
  n217 = Release Queue(queue=w3) -> ()  [unwired: 2 in, 3 out]
  n218 = Unregister For Events(event registration refnum=w34, error in=w39) -> (error out=w35:errorcluster)
  n219 = Close Reference(reference=w24) -> ()  [unwired: 1 in, 1 out]
  n220 = Release Queue(queue=w1) -> ()  [unwired: 2 in, 3 out]
  n221 = Merge Errors(w35, w2, w7, w26) -> (w38:errorcluster)
  n222 = call "Destroy User Event - Stop.vi"("error in (no error)"=w38, "User Event - Stop"=w36) -> ()  [unwired: 9 in, 1 out]
